vi "Destroy.vi"(8 "error in (no error)":errorcluster, 11 "StringList in":refnum<class "StringList.lvclass">) -> (0 "error out":errorcluster)   [LabVIEW 2013, in "LapDog.Collections.v1.Lists.lvlib" / "StringList.lvclass"]
uses:
  StringList.lvclass
  StringList.lvclass/StringList.ctl
  ObjectList/ObjectList.lvclass
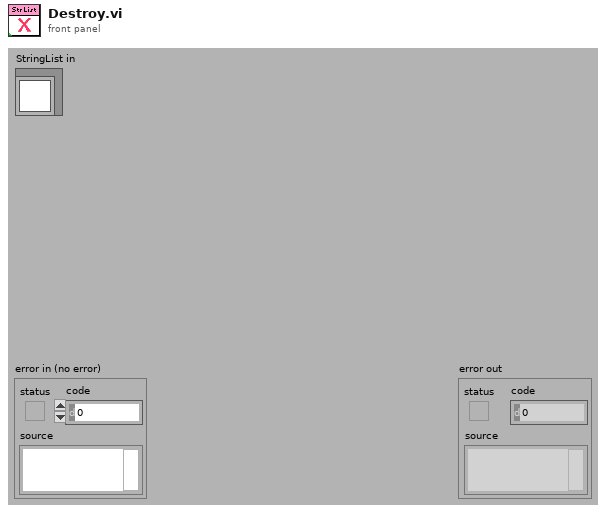
[diagram p1: front panel]
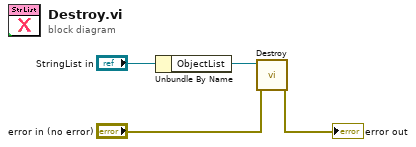
[diagram p0: block diagram]
diagram:
  n1 = Unbundle By Name("StringList in") -> ("ObjectList"=w3:refnum<class "ObjectList.lvclass">)
  n2 = call-dynamic "Destroy.vi"("error in (no error)"="error in (no error)", "List in"=w3) -> ("error out"=→"error out":errorcluster)  [unwired: 9 in]
